vi "Climb Controller.vi"(8 "error in":errorcluster) -> ()   [LabVIEW 2016]
doc: "This VI executes continuously carrying out the current operation and responding to updates or new operations. It will often contain the timing or control code that is difficult to place directly in TeleOp. This VI generally opens all sensors and motors and isolates the rest of the robot code from knowing how the operations are carried out."
uses:
  Climb Setpoints.ctl
  Climb Operations.ctl
  <vilib>/Rock Robotics/SystemInterfaces/DIO/FPGA_DIOPWMChannel.ctl
  <vilib>/Rock Robotics/WPI/SafetyOutput/WPI_SafetyOutputConfigMenu.ctl
  <vilib>/Rock Robotics/WPI/MotorControl/WPI_MotorControlOpen SPARK.vi
  <vilib>/Rock Robotics/Network Tables/NT Write Boolean.vi
panel:
  out "Current\nCmd":string
  # "Tip: It may be helpful to observe inputs and sensor values.\nYou may also want to display tuning or debugging controls."
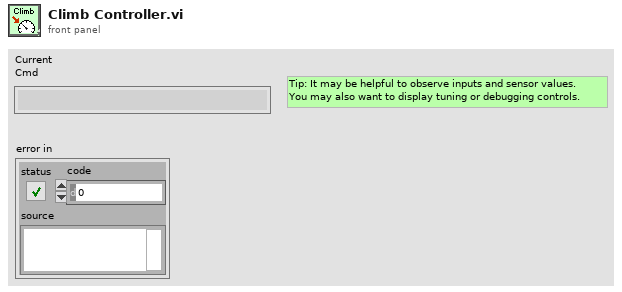
[diagram p1: front panel]
types:
  T1 = typedef "WPI_SafetyOutputConfigMenu.ctl" = enum16{"Enable", "Disable"}
  T2 = typedef "FPGA_DIOPWMChannel.ctl" = enum8{"PWM 0", "PWM 1", "PWM 2", "PWM 3", "PWM 4", "PWM 5", "PWM 6", "PWM 7", "PWM 8", "PWM 9", "PWM MXP 0", "PWM MXP 1", "PWM MXP 2", "PWM MXP 3", "PWM MXP 4", "PWM MXP 5", "PWM MXP 6", "PWM MXP 7", "PWM MXP 8", "PWM MXP 9", "Invalid"}
  T3 = typedef "Climb Setpoints.ctl" = cluster{"Operation":T4, "Setpoint":dbl, "Duration":dbl}
  T4 = typedef "Climb Operations.ctl" = enum16{"Reserve", "Read Current", "Immediate", "Climb"}
  T5 = typedef "WPI_MotorControlDeviceRef.ctl" = cluster{"DeviceStatus":errorcluster, "Type":T6, "PWM":cluster{"PWM Channel":T2, "DeadBand":T7}, "CAN":cluster{"Device Number":u8, "SetOutput VI Ref":variant, "GetOutput VI Ref":variant, "Enable VI Ref":variant, "Disable VI Ref":variant, "Data":variant}, "Invert":bool}
  T6 = typedef "WPI_MotorControlType.ctl" = enum16{"PWM", "CAN"}
  T7 = typedef "WPI_PWMDeadband.ctl" = cluster{"Name":string, "maxPositivePwm":i32, "minPositivePwm":i32, "centerPwm":i32, "maxNegativePwm":i32, "minNegativePwm":i32, "angularRange":u16}
  T8 = typedef "Command Status Info.ctl" = cluster{"Name":string, "Status":T9, "notifier out":T10}
  T9 = typedef "Completion Status.ctl" = enum16{"Successful", "Aborted", "Incomplete"}
  T10 = typedef "Completion Notifier.ctl" = refnum<notifier>
  T11 = cluster{"Default Command":T3, "Command Timing":cluster{"Start Time (ms)":u32, "Iterations":i32}, "Command Arguments":cluster{"Command Info":T8, "Description":string, "Default Command":T3, "notifier out":refnum<notifier>, "Subsystem Name":string}}
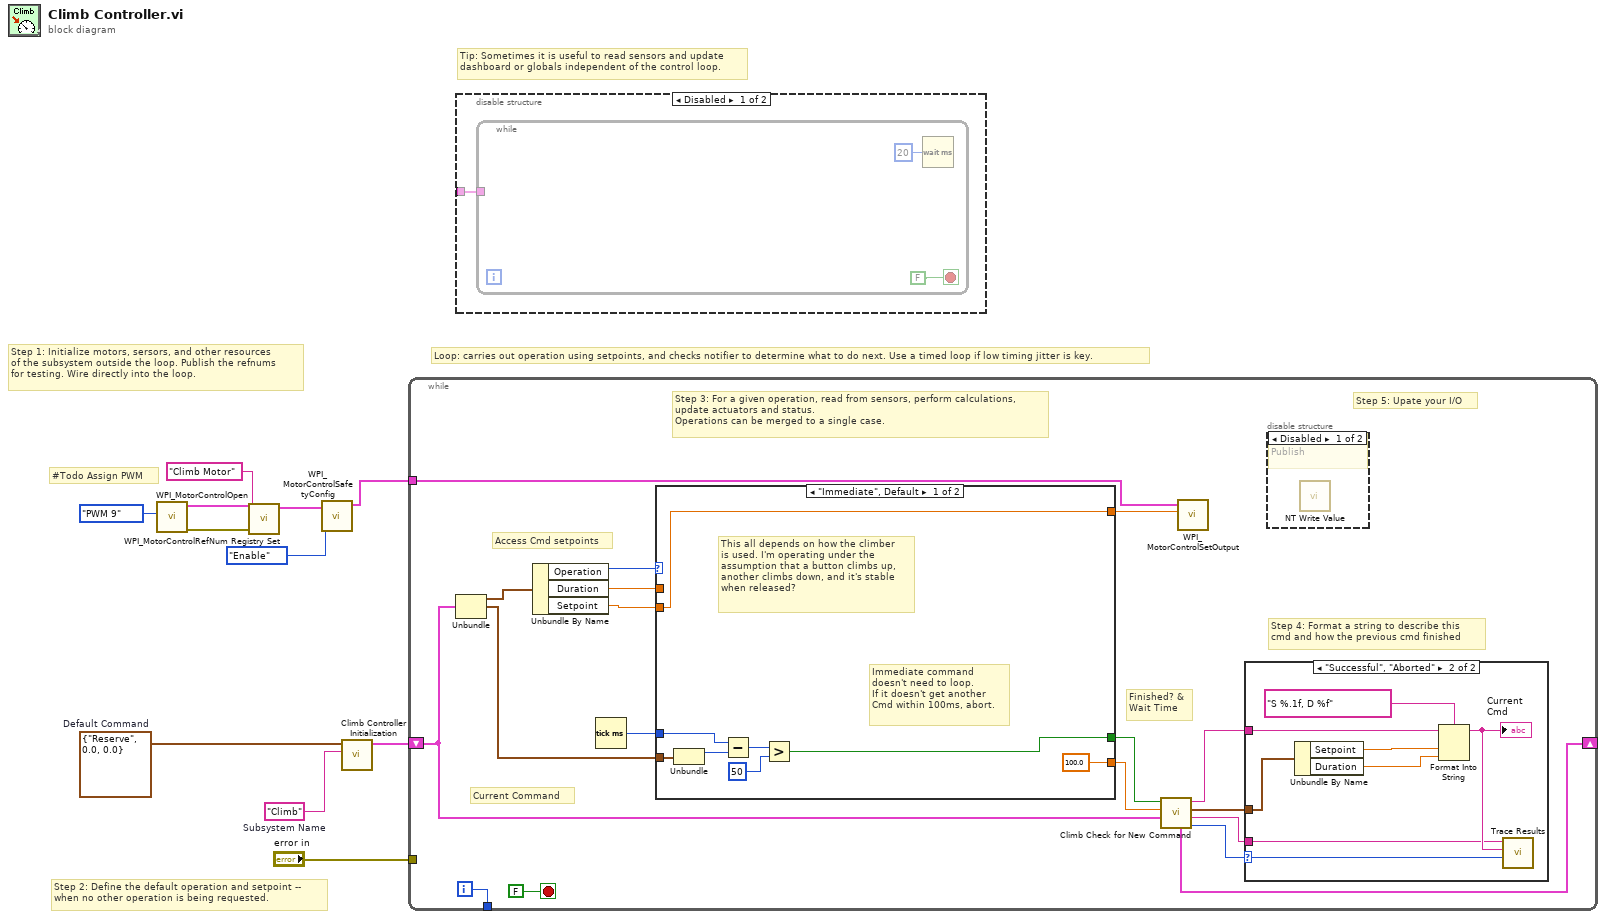
[diagram p0: block diagram]
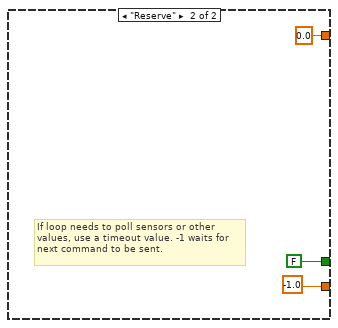
[diagram p5: hidden frame]
diagram:
  w8 = T3 {"Operation"=enum."Reserve", "Setpoint"=0.0, "Duration"=0.0}  # Default Command
  w9 = "Climb"  # Subsystem Name
  # "#Todo Assign PWM"
  # "Tip: Sometimes it is useful to read sensors and update\ndashboard or globals independent of the control loop."
  # "Step 2: Define the default operation and setpoint --\nwhen no other operation is being requested."
  # "Step 1: Initialize motors, sersors, and other resources\nof the subsystem outside the loop. Publish the refnums\nfor testing. Wire directly into the loop."
  # "Loop: carries out operation using setpoints, and checks notifier to determine what to do next. Use a timed loop if low timing jitter is key."
  n1 = call-poly <vilib>:"WPI_MotorControlOpen.vi"("PWM Channel"=FPGA_DIOPWMChannel."PWM 9") -> ("error out"=w2:errorcluster, "MotorControlDeviceRef"=w6:T5)  [unwired: 9 in]
  n2 = call <vilib>:"WPI_MotorControlRefNum Registry Set.vi"("error in (no error)"=w2, "refnum name"="Climb Motor", "MotorControlDevRef"=w6) -> ("MotorControlDevRef"=w4:T5)  [unwired: 7 in, 1 out]
  n3 = call <vilib>:"WPI_MotorControlSafetyConfig.vi"("mode"=WPI_SafetyOutputConfigMenu."Enable", "MotorControlDevRef"=w4) -> ("MotorControlDevRef"=w1:T5)  [unwired: 8 in, 1 out]
  n4 = call "Climb Controller Initialization.vi"("Subsystem Name"=w9, "Default Command"=w8) -> ("Command Info"=w10:T11)  [unwired: 9 in]
  n5 = while {
    shift-right: [w20] -> _
    shift-left: w10 -> [w21]
    tunnel: [w28] -> _
    tunnel: "error in" -> [_]
    tunnel: w1 -> [w13]
    i -> [w28]
    stop <- FALSE stop-if-true
    # "Step 5: Upate your I/O"
    # "Step 4: Format a string to describe this\ncmd and how the previous cmd finished"
    # "Current Command"
    # "Access Cmd setpoints"
    # "Finished? &\nWait Time"
    # "Step 3: For a given operation, read from sensors, perform calculations,\nupdate actuators and status.\nOperations can be merged to a single case."
    n6 = Unbundle(w21) -> ("Default Command"=w27:T3, "Command Timing"=w23:cluster{"Start Time (ms)":u32, "Iterations":i32})  [unwired: 1 out]
    n7 = Unbundle By Name(w27) -> ("Operation"=w26:T4, "Duration"=w25:dbl, "Setpoint"=w22:dbl)
    n8 = Tick Count (ms)() -> (millisecond timer value=w24:u32)
    n9 = case shown="\"Immediate\", Default" w26 {
      tunnel: [100.0 -1.0] -> w18
      tunnel: [w39 FALSE ("ignore previous (F)")] -> w19
      tunnel: w23 -> [w41 _]
      tunnel: w25 -> [_ _]
      tunnel: w24 -> [w40 _]
      tunnel: w22 -> [w38 _]
      tunnel: [w38 0.0 ("Setpoint")] -> w12
      frame "Immediate", Default {
        # "This all depends on how the climber\nis used. I'm operating under the\nassumption that a button climbs up,\nanother climbs down, and it's stable\nwhen released?"
        # "Immediate command\ndoesn't need to loop.\nIf it doesn't get another\nCmd within 100ms, abort."
        n10 = Unbundle(w41) -> ("Start Time (ms)"=w44:u32)  [unwired: 1 out]
        n11 = Subtract(x=w40, y=w44) -> (x-y=w43:u32)
        n12 = Greater?(x=w43, y=u8 50 ("Left Motor")) -> (0:w39:bool)
      }
      frame "Reserve" {
        # "If loop needs to poll sensors or other\nvalues, use a timeout value. -1 waits for\nnext command to be sent."
      }
    }
    n13 = call "Climb Check for New Command.vi"("Current Command"=w21, "Wait time (ms)"=w18, "Finished?"=w19) -> ("Completion"=w14:T9, "Subsystem Name"=w15:string, "Current Command"=w16:T3, "Initial Trace String"=w17:string, "NextCommand"=w20:T11)  [unwired: 4 in]
    n14 = call <vilib>:"WPI_MotorControlSetOutput.vi"("Output"=w12, "MotorControlDevRef"=w13) -> ()  [unwired: 7 in, 3 out]
    n15 = case shown="\"Successful\", \"Aborted\"" w14 {
      selector: w14 -> [_ w37]
      tunnel: w17 -> [_ w33]
      tunnel: w16 -> [_ w34]
      tunnel: w15 -> [_ w30]
      frame "Incomplete", Default {
        # "Continuing current command"
      }
      frame "Successful", "Aborted" {
        # "Report and setup for next command"
        n16 = Unbundle By Name(w34) -> ("Setpoint"=w36:dbl, "Duration"=w31:dbl)
        n17 = Format Into String(format string="S %.1f, D %f", initial string=w33, w36, w31) -> (resulting string=w32:string)  [unwired: 1 in, 1 out]
        "Current\nCmd" <- w32
        n18 = call <vilib>:"Trace Results.vi"("Status of previous command"=w37, "Description"=w32, "Subsystem"=w30) -> ()  [unwired: 9 in]
      }
    }
    n19 = disable-structure shown="Disabled" {
      frame Disabled {
        # "Publish"
        n20 = call-poly <vilib>:"NT Write Value.vi"() -> ()  [unwired: 11 in, 1 out]
      }
      frame Enabled {
      }
    }
  }
  n21 = disable-structure shown="Disabled" {
    disable-tunnel: _ -> [w49 _]
    frame Disabled {
      n22 = while {
        tunnel: w49 -> [_]
        stop <- FALSE stop-if-true
        n23 = Wait (ms)(milliseconds to wait=u32 20) -> ()  [unwired: 1 out]
      }
    }
    frame Enabled {
    }
  }
